vi "ReadWriteTopicData.vi"(3 "error in (no error)":errorcluster, 4 "timeout ms (1000)":i32=1000, 5 "connection ID in":refnum<k5>) -> (0 "error out":errorcluster, 1 "data out":string, 2 "connection ID out":refnum<k5>)   [LabVIEW 2012]
uses:
  parsing/std_msgs/subs/parse_u32_scalar.vi
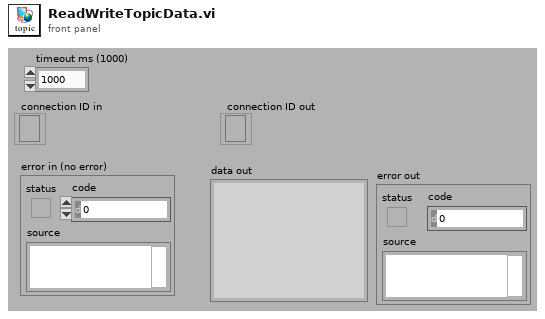
[diagram p1: front panel]
types:
  T1 = enum16{"Standard", "Buffered", "CRLF", "Immediate"}
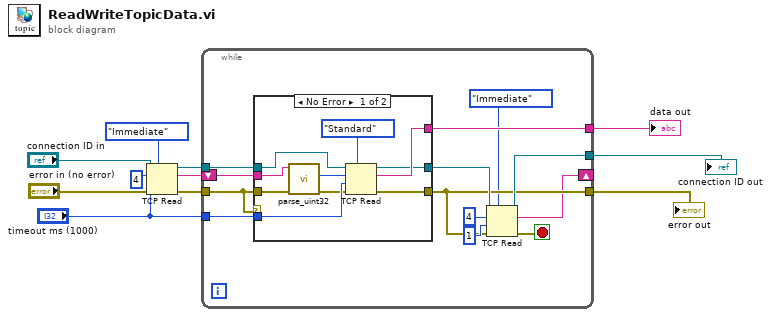
[diagram p0: block diagram]
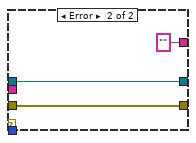
[diagram p2: hidden frame]
diagram:
  n1 = TCP Read(connection ID="connection ID in", bytes to read=4, error in (no error)="error in (no error)", 7:T1."Immediate" ("mode (standard)"), 9:"timeout ms (1000)") -> (connection ID out=w7:refnum<k5>, data out=w4:string, error out=w3:errorcluster)
  n2 = while {
    tunnel: [w24] -> w11
    tunnel: [w15] -> w10
    tunnel: w7 -> [w23]
    tunnel: w3 -> [w21]
    tunnel: "timeout ms (1000)" -> [w20]
    tunnel: [w16] -> w1
    shift-right: [w13] -> _
    shift-left: w4 -> [w22]
    stop <- w14 stop-if-true
    n3 = case shown="No Error" w21 {
      tunnel: [w34 "" ("data out")] -> w24
      tunnel: [w33 w36] -> w15
      tunnel: [w32 w37] -> w19
      tunnel: w21 -> [w27 w36]
      tunnel: w23 -> [w31 w37]
      tunnel: w22 -> [w25 _]
      tunnel: w20 -> [w29 _]
      frame No Error {
        n4 = call-poly "parse_uint32.vi"("error in"=w27, "msg in"=w25) -> ("error out"=w26:errorcluster, "number"=w28:u32)  [unwired: 3 in, 1 out]
        n5 = TCP Read(connection ID=w31, bytes to read=w28, error in (no error)=w26, 7:T1."Standard" ("mode (standard)"), 9:w29) -> (connection ID out=w32:refnum<k5>, data out=w34:string, error out=w33:errorcluster)
      }
      frame Error {
      }
    }
    n6 = TCP Read(connection ID=w19, bytes to read=4, error in (no error)=w15, 7:T1."Immediate" ("mode (standard)"), 9:1 ("timeout ms (25000)")) -> (connection ID out=w16:refnum<k5>, data out=w13:string, error out=w14:errorcluster)
  }
  "data out" <- w11
  "error out" <- w10
  "connection ID out" <- w1
